vi "UsrProfiles-Select specified user.vi"(8 "error in (no error)":errorcluster, 11 "New user name":string) -> (0 "error out":errorcluster)   [LabVIEW 2020]
uses:
  Globals/gl_UsrProfiles globals.vi
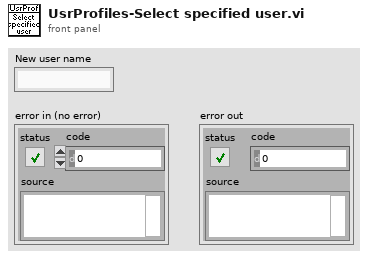
[diagram p1: front panel]
types:
  T1 = typedef "User login window refs.ctl" = cluster{"User profiles window ref":refnum<k9>, "Users listbox":refnum<vi>, "Profiles listbox":refnum<vi>, "Last used":refnum<vi>}
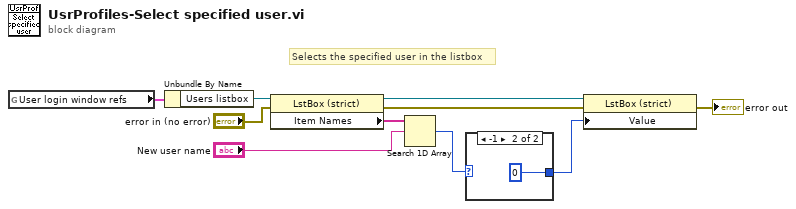
[diagram p0: block diagram]
diagram:
  # "Selects the specified user in the listbox"
  n1 = global read "gl_UsrProfiles globals.vi" "User login window refs"() -> (w10:T1)
  n2 = Unbundle By Name(w10) -> ("Users listbox"=w3:refnum<vi>)
  n3 = property on="Property Node" class="LstBox (strict)"(reference=w3, error in="error in (no error)") -> (reference out=w6:refnum<vi>, error out=w8:errorcluster, "Item Names"=w4:string[])
  n4 = Search 1D Array(1D array=w4, element="New user name") -> (index of element=w2:i32)  [unwired: 1 in]
  n5 = case shown="-1" w2 {
    selector: w2 -> [w11 _]
    tunnel: [w11 0 ("index of element")] -> w1
    frame Default {
    }
    frame -1 {
    }
  }
  n6 = property on="Property Node" class="LstBox (strict)"(reference=w6, error in=w8, "Value"=w1) -> (error out=→"error out":errorcluster)  [unwired: 1 out]
